vi "LiCor_data_txt_to_array.vi"(1 "LiCor data string":string) -> (0 "Array":dbl[](array[numeric]))   [LabVIEW 2010]
panel:
  # "LiCar Data Text to Array\n\nThis VI converts the text data sent by the LiCor instrument into an \narray of values."
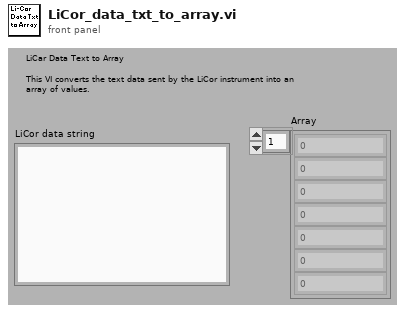
[diagram p1: front panel]
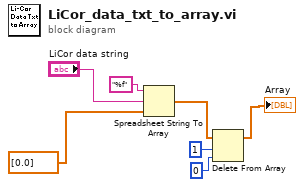
[diagram p0: block diagram]
diagram:
  n1 = Spreadsheet String To Array(format string="%f", spreadsheet string="LiCor data string", array type (2D Dbl)=dbl[] [0.0] ("Array 2")) -> (array=w2:dbl[])  [unwired: 1 out]
  n2 = Delete From Array(array=w2, length=1, index=0) -> (array with subset deleted=→"Array":dbl[])  [unwired: 1 out]
